vi "Object To Pretty String.vi"(6 "pretty print? (T)":bool=TRUE, 7 "enable LabVIEW extensions? (T)":bool=TRUE, 8 "error in (no error)":errorcluster, 11 "JSON Value in":refnum<class "JSON Value.lvclass">) -> (0 "error out":errorcluster, 3 "Pretty Print String":string)   [LabVIEW 2016, in "JSON Value.lvclass"]
doc: "Pretty prints the given JSON data in an easier to read format."
uses:
  JSON Helper/JSON Value.lvclass
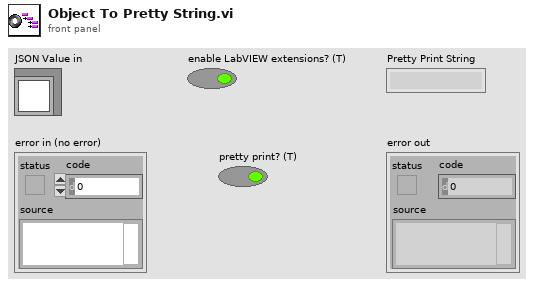
[diagram p1: front panel]
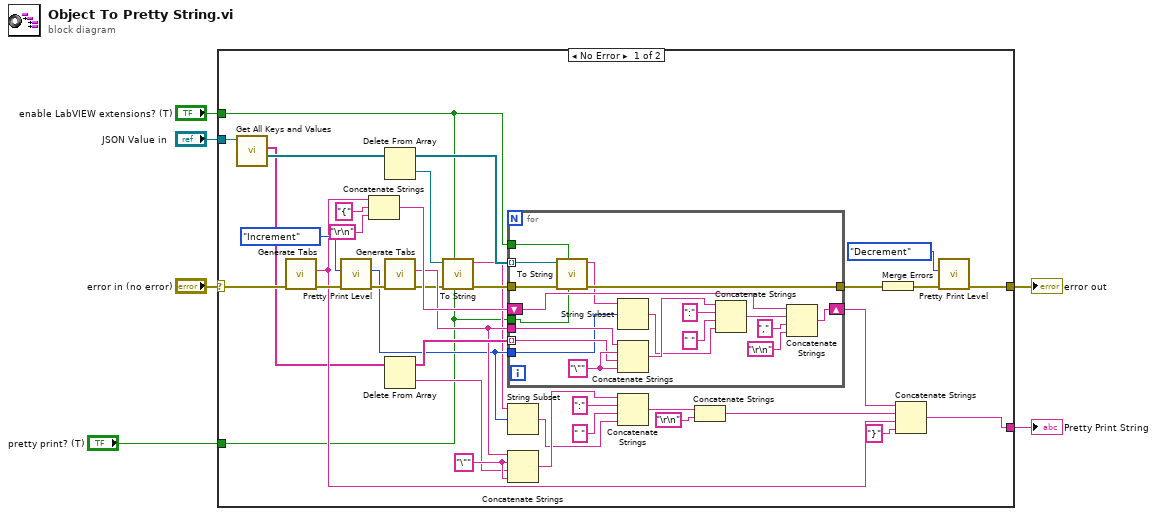
[diagram p0: block diagram]
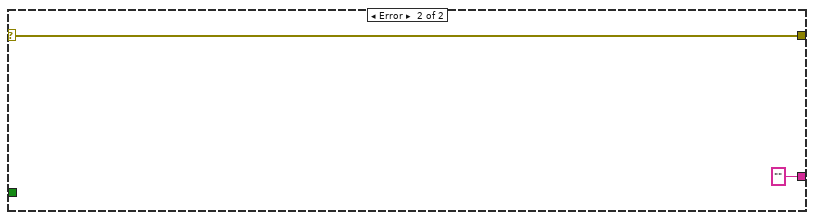
[diagram p2: hidden frame]
diagram:
  n1 = case shown="No Error" "error in (no error)" {
    selector: "error in (no error)" -> [w27 w63]
    tunnel: [w29 ""] -> w6
    tunnel: [w28 w63] -> w5
    tunnel: "JSON Value in" -> [w18 _]
    tunnel: "enable LabVIEW extensions? (T)" -> [w8 _]
    tunnel: "pretty print? (T)" -> [w7 _]
    frame No Error {
      w23 = "\"" ("string")
      n2 = call "Get All Keys and Values.vi"("JSON Value in"=w18) -> ("values"=w26:refnum<class "JSON Value.lvclass">[], "keys"=w25:string[])  [unwired: 8 in, 1 out]
      n3 = call "Generate Tabs.vi"("error in (no error)"=w27) -> ("error out"=w40:errorcluster, "Tabs"=w30:string)  [unwired: 9 in]
      n4 = call "Pretty Print Level.vi"("error in (no error)"=w40, "Action"=enum16{"Increment", "Decrement", "Get", "Reset"}."Increment") -> ("error out"=w37:errorcluster, "Numeric"=w11:i32)  [unwired: 8 in]
      n5 = Concatenate Strings(w30, "{" ("string"), "\r\n") -> (w41:string)
      n6 = Delete From Array(array=w26) -> (deleted portion=w14:refnum<class "JSON Value.lvclass">, array with subset deleted=w36:refnum<class "JSON Value.lvclass">[])  [unwired: 2 in]
      n7 = call "Generate Tabs.vi"("error in (no error)"=w37) -> ("error out"=w13:errorcluster, "Tabs"=w16:string)  [unwired: 9 in]
      n8 = Delete From Array(array=w25) -> (deleted portion=w21:string, array with subset deleted=w19:string[])  [unwired: 2 in]
      n9 = call "To String.vi"("pretty print? (T)"=w7, "enable LabVIEW extensions? (T)"=w8, "error in (no error)"=w13, "JSON Value in"=w14) -> ("error out"=w12:errorcluster, "String"=w10:string)  [unwired: 6 in]
      n10 = for {
        tunnel: w36 -> [w50] mode=indexing
        shift-right: [w60] -> w34
        shift-left: w41 -> [w59]
        tunnel: w16 -> [w52]
        tunnel: w19 -> [w55] mode=indexing
        tunnel: w12 -> [w51]
        tunnel: [w49] -> w15
        tunnel: w11 -> [w47]
        tunnel: w8 -> [w45]
        tunnel: w7 -> [w44]
        w57 = "\"" ("string")
        n11 = call "To String.vi"("pretty print? (T)"=w44, "enable LabVIEW extensions? (T)"=w45, "error in (no error)"=w51, "JSON Value in"=w50) -> ("error out"=w49:errorcluster, "String"=w48:string)  [unwired: 6 in]
        n12 = String Subset(string=w48, offset (0)=w47) -> (substring=w46:string)  [unwired: 1 in]
        n13 = Concatenate Strings(w52, w57, w55, w57) -> (w58:string)
        n14 = Concatenate Strings(w58, ":" ("string"), " " ("string"), w46) -> (w54:string)
        n15 = Concatenate Strings(w59, w54, "," ("string"), "\r\n") -> (w60:string)
      }
      n16 = String Subset(string=w10, offset (0)=w11) -> (substring=w9:string)  [unwired: 1 in]
      n17 = Concatenate Strings(w16, w23, w21, w23) -> (w22:string)
      n18 = Concatenate Strings(w22, ":" ("string"), " " ("string"), w9) -> (w20:string)
      n19 = Concatenate Strings(w20, "\r\n") -> (w33:string)
      n20 = Merge Errors(w15) -> (w39:errorcluster)
      n21 = Concatenate Strings(w34, w33, w30, "}" ("string")) -> (w29:string)
      n22 = call "Pretty Print Level.vi"("error in (no error)"=w39, "Action"=enum16{"Increment", "Decrement", "Get", "Reset"}."Decrement") -> ("error out"=w28:errorcluster)  [unwired: 8 in, 1 out]
    }
    frame Error {
    }
  }
  "error out" <- w5
  "Pretty Print String" <- w6
